vi "pressure_unit_converter.vi"(1 "Output Unit":string(combo), 2 "Input":dbl[](array[numeric]) format="%#_13g", 3 "Input Unit":string(combo)) -> (0 "Output":dbl[](array[numeric]))   [LabVIEW 2017, in "sensor_translation.lvlib"]
uses:
  sensor_translation.lvlib
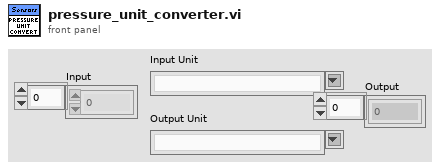
[diagram p1: front panel]
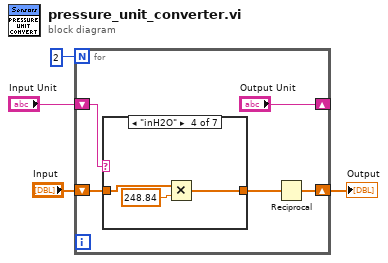
[diagram p0: block diagram]
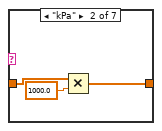
[diagram p3: hidden frame]
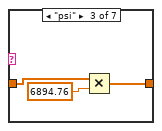
[diagram p4: hidden frame]
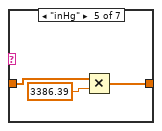
[diagram p5: hidden frame]
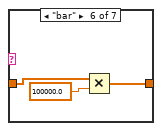
[diagram p6: hidden frame]
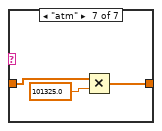
[diagram p7: hidden frame]
diagram:
  n1 = for {
    N: 2 -> [_]
    shift-right: ["Output Unit"] -> _
    shift-left: "Input Unit" -> [w9]
    shift-right: [w5] -> w1
    shift-left: "Input" -> [w8]
    n2 = case shown="\"inH2O\"" w9 {
      tunnel: w8 -> [w10 w12 w16 w19 w22 w25 w28]
      tunnel: [w10 w13 w14 w17 w20 w23 w26] -> w6
      frame "Pa", Default {
        # "First convert to Pascal"
      }
      frame "kPa" {
        n3 = Multiply(x=w12, y=1000.0) -> (x*y=w13:dbl[])
      }
      frame "psi" {
        n4 = Multiply(x=w16, y=6894.76) -> (x*y=w14:dbl[])
      }
      frame "inH2O" {
        n5 = Multiply(x=w19, y=248.84) -> (x*y=w17:dbl[])
      }
      frame "inHg" {
        n6 = Multiply(x=w22, y=3386.39) -> (x*y=w20:dbl[])
      }
      frame "bar" {
        n7 = Multiply(x=w25, y=100000.0) -> (x*y=w23:dbl[])
      }
      frame "atm" {
        n8 = Multiply(x=w28, y=101325.0) -> (x*y=w26:dbl[])
      }
    }
    n9 = Reciprocal(x=w6) -> (1/x=w5:dbl[])
  }
  "Output" <- w1
